vi "HW3_2017_WMA.vi"() -> ()   [LabVIEW 2018]
uses:
  <vilib>/sound2/lvsound2.llb/Sound Output Task ID.ctl
panel:
  in  "shut up":bool
  out "Boolean 3":bool
  out "Boolean 2":bool
  out "Cluster 2":T1
  out "Cluster 3":T1
  out "Cluster 4":T1
  out "Cluster 5":T1
  out "Cluster 6":T1
  out "Cluster 7":T1
  in  "START/STOP/CLEAR":bool
  in  "min":dbl
  in  "hour":dbl
  in  "OK Button":bool
  out "Boolean":bool
  in  "SET ALARM":bool
  out "ALARMING TIME":string
  out "DATE":string
  in  "reinstate":bool
  in  "sec":dbl
  in  "min":dbl
  in  "hour":dbl
  in  "reset":bool
  out "sec":dbl(knob) scale=0.0..60.0
  out "min":dbl(knob) scale=0.0..60.0
  out "hour":dbl(knob) scale=0.0..12.0
  in  "stop":bool
  in  "OK Button 3":bool
  in  "Path 2":path
  out "new picture":picture
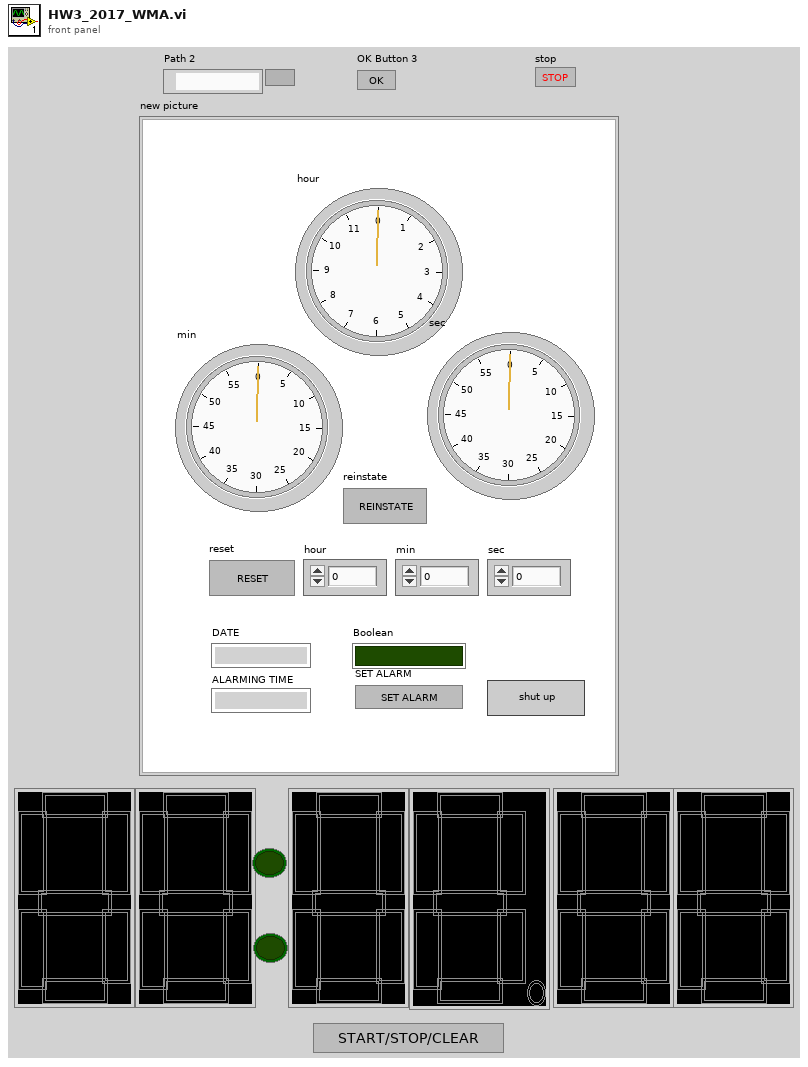
[diagram p1: front panel]
types:
  T1 = cluster{"0":bool, "1":bool, "2":bool, "3":bool, " 4":bool, "5":bool, "6":bool, "p":bool}
  T2 = cluster{"0":bool, "1":bool, "2":bool, "3":bool, " 4":bool, "5":bool, "6":bool, "p":bool}[]
  T3 = typedef "LVDateTimeRec.ctl" = cluster{"fractional second":dbl, "second":i32, "minute":i32, "hour":i32, "day of month":i32, "month":i32, "year":i32, "day of week":i32, "day of year":i32, "DST":i32}
  T4 = typedef "Sound Output Task ID.ctl" = u32
  T5 = typedef "imagedata.ctl" = cluster{"image type":i32, "image depth":i32, "image":u8[], "mask":u8[], "colors":u32[], "Rectangle":cluster{"left":i16, "top":i16, "right":i16, "bottom":i16}}
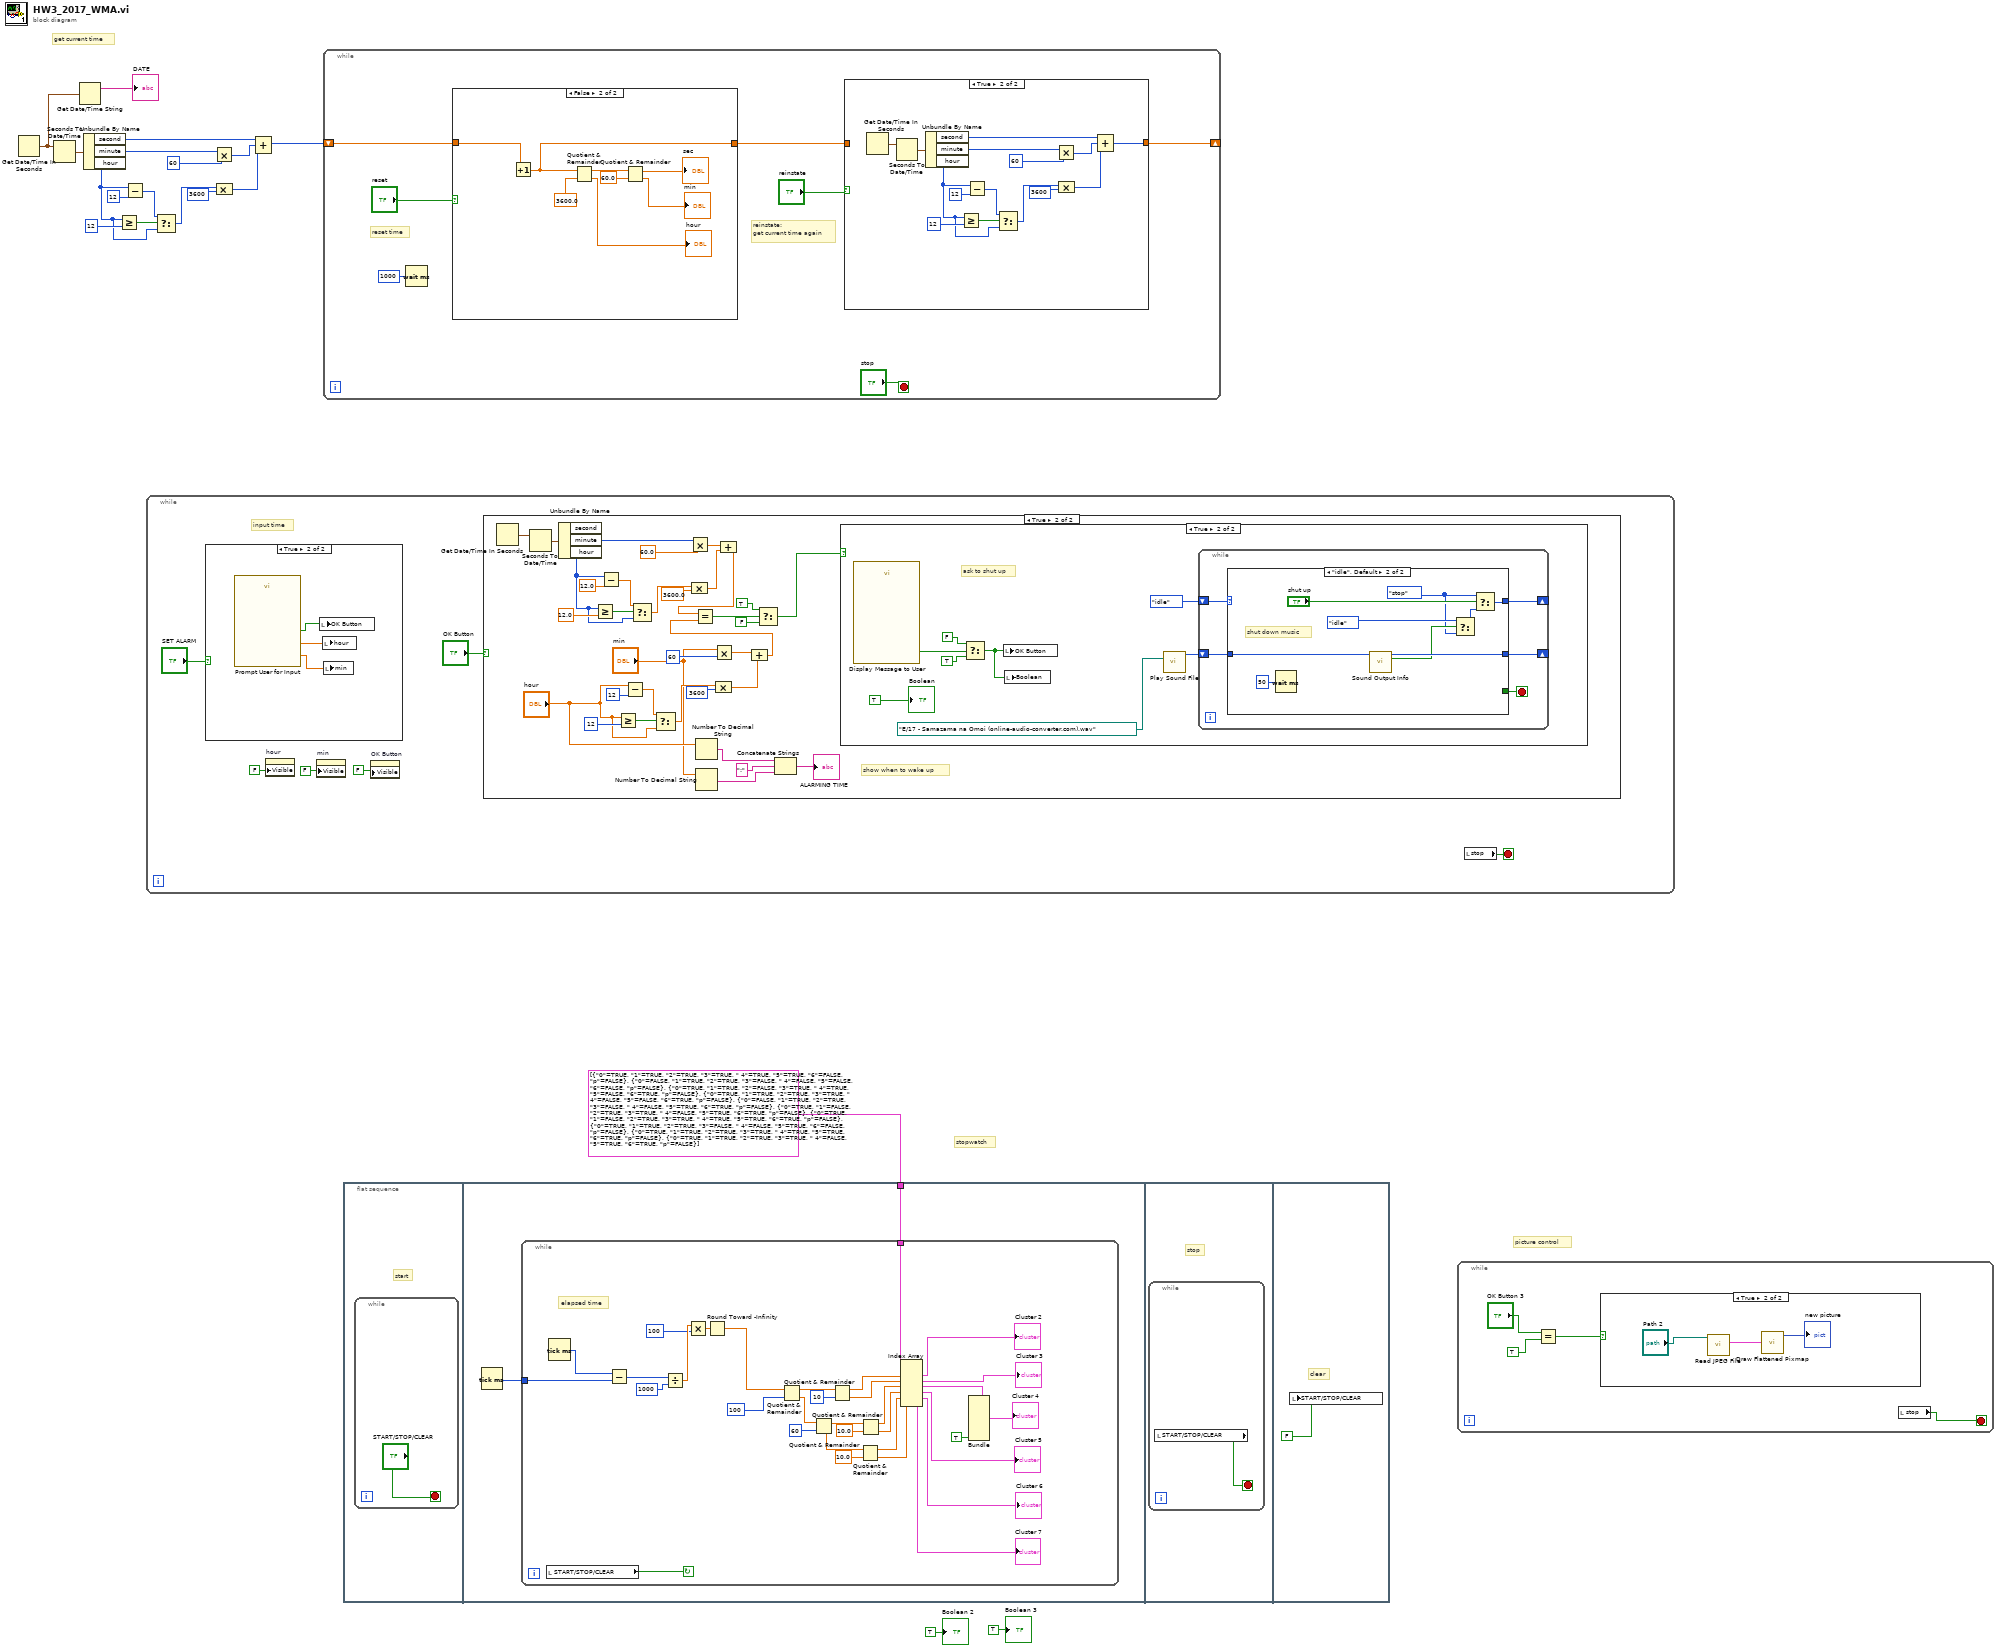
[diagram p0: block diagram]
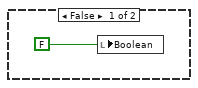
[diagram p4: hidden frame]
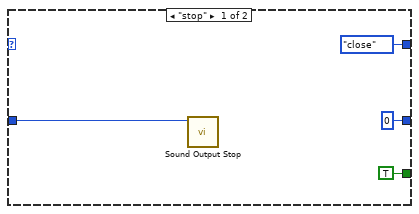
[diagram p5: hidden frame]
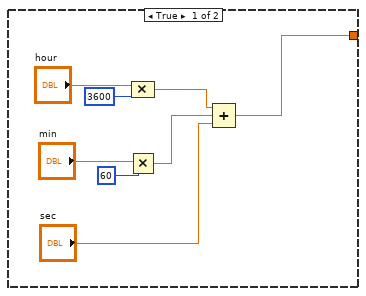
[diagram p8: hidden frame]
diagram:
  # "get current time"
  # "stopwatch"
  # "picture control"
  n1 = Get Date/Time In Seconds() -> (seconds since 1Jan1904=w8:timestamp)
  n2 = Seconds To Date/Time(time stamp (now)=w8) -> (date time rec=w17:T3)  [unwired: 1 in]
  n3 = Get Date/Time String(seconds (now)=w8) -> (date string=→"DATE":string)  [unwired: 2 in, 1 out]
  n4 = Unbundle By Name(w17) -> ("second"=w15:i32, "minute"=w16:i32, "hour"=w10:i32)
  n5 = Greater Or Equal?(x=w10, y=12) -> (x >= y?=w13:bool)
  n6 = Subtract(x=w10, y=12) -> (x-y=w11:i32)
  n7 = while {
    stop <- w21 stop-if-true
    # "input time"
    n8 = case shown="True" "SET ALARM" {
      frame False {
      }
      frame True {
        n9 = call "Prompt User for Input"() -> ("Minute"=w89:dbl, "Hour"=w88:dbl, "OK"=w87:bool)  [unwired: 16 in, 1 out]
        n10 = local write "OK Button"(w87) -> ()
        n11 = local write "hour"(w88) -> ()
        n12 = local write "min"(w89) -> ()
      }
    }
    n13 = property on="hour" class="DigNum (strict)"("Visible"=FALSE) -> ()  [unwired: 2 in, 2 out]
    n14 = property on="min" class="DigNum (strict)"("Visible"=FALSE) -> ()  [unwired: 2 in, 2 out]
    n15 = property on="OK Button" class="Bool (strict)"("Visible"=FALSE) -> ()  [unwired: 2 in, 2 out]
    n16 = case shown="True" "OK Button" {
      frame False {
      }
      frame True {
        # "show when to wake up"
        n17 = Get Date/Time In Seconds() -> (seconds since 1Jan1904=w29:timestamp)
        n18 = Seconds To Date/Time(time stamp (now)=w29) -> (date time rec=w32:T3)  [unwired: 1 in]
        n19 = Unbundle By Name(w32) -> ("minute"=w33:i32, "hour"=w27:i32)  [unwired: 1 out]
        n20 = Greater Or Equal?(x=w27, y=12.0) -> (x >= y?=w35:bool)
        n21 = Subtract(x=w27, y=12.0) -> (x-y=w37:dbl)
        n22 = Greater Or Equal?(x="hour", y=12) -> (x >= y?=w54:bool)
        n23 = Subtract(x="hour", y=12) -> (x-y=w52:dbl)
        n24 = Select(t=w37, s=w35, f=w27) -> (s? t:f=w38:dbl)
        n25 = Select(t=w52, s=w54, f="hour") -> (s? t:f=w51:dbl)
        n26 = Multiply(x=w33, y=60.0) -> (x*y=w39:dbl)
        n27 = Compound Arithmetic op=MULTIPLY(w38, 3600.0) -> (w40:dbl)
        n28 = Number To Decimal String(number="hour") -> (decimal integer string=w46:string)  [unwired: 1 in]
        n29 = Number To Decimal String(number="min") -> (decimal integer string=w44:string)  [unwired: 1 in]
        n30 = Multiply(x="min", y=60) -> (x*y=w57:dbl)
        n31 = Compound Arithmetic op=MULTIPLY(w51, 3600) -> (w56:dbl)
        n32 = Compound Arithmetic op=ADD(w39, w40) -> (w28:dbl)
        n33 = Compound Arithmetic op=ADD(w57, w56) -> (w50:dbl)
        n34 = Equal?(x=w28, y=w50) -> (x = y?=w49:bool)
        n35 = Select(t=TRUE, s=w49, f=FALSE) -> (s? t:f=w26:bool)
        n36 = Concatenate Strings(w46, ":", w44) -> (→"ALARMING TIME":string)
        n37 = case shown="True" w26 {
          frame False {
            n38 = local write "Boolean"(FALSE ("Boolean")) -> ()
          }
          frame True {
            # "ask to shut up"
            n39 = call "Display Message to User"() -> ("OK"=w66:bool)  [unwired: 10 in, 1 out]
            n40 = Select(t=FALSE ("Boolean"), s=w66, f=TRUE) -> (s? t:f=w64:bool)
            n41 = local write "OK Button"(w64) -> ()
            n42 = local write "Boolean"(w64) -> ()
            n43 = call <vilib>:"Play Sound File.vi"("path"=path "E:/17 - Samazama na Omoi (online-audio-converter.com).wav" ("Path")) -> ("task ID"=w62:T4)  [unwired: 9 in, 1 out]
            n44 = while {
              shift-right: [w69] -> _
              shift-left: enum16{"start", "stop", "close", "idle"}."idle" -> [w73]
              shift-right: [w71] -> _
              shift-left: w62 -> [w70]
              stop <- w72 stop-if-true
              n45 = case shown="\"idle\", Default" w73 {
                tunnel: [TRUE _] -> w72
                tunnel: [T4 0 ("task ID") w84] -> w71
                tunnel: w70 -> [w77 w85]
                tunnel: [enum16{"start", "stop", "close", "idle"}."close" w79] -> w69
                frame "stop" {
                  n46 = call <vilib>:"Sound Output Stop.vi"("task ID"=w77) -> ()  [unwired: 9 in, 2 out]
                }
                frame "idle", Default {
                  w78 = enum16{"start", "stop", "close", "idle"}."stop"
                  # "shut down music"
                  n47 = Wait (ms)(milliseconds to wait=u32 50) -> ()  [unwired: 1 out]
                  n48 = call <vilib>:"Sound Output Info.vi"("task ID"=w85) -> ("is playing?"=w83:bool, "task ID out"=w84:T4)  [unwired: 7 in, 2 out]
                  n49 = Select(t=enum16{"start", "stop", "close", "idle"}."idle", s=w83, f=w78) -> (s? t:f=w81:enum16{"start", "stop", "close", "idle"})
                  n50 = Select(t=w78, s="shut up", f=w81) -> (s? t:f=w79:enum16{"start", "stop", "close", "idle"})
                }
              }
            }
            "Boolean" <- TRUE ("Boolean")
          }
        }
      }
    }
    n51 = local read "stop"() -> (w21:bool)
  }
  n52 = Select(t=w11, s=w13, f=w10) -> (s? t:f=w9:i32)
  n53 = Multiply(x=w16, y=60) -> (x*y=w5:i32)
  n54 = Compound Arithmetic op=MULTIPLY(w9, 3600) -> (w4:i32)
  n55 = Compound Arithmetic op=ADD(w15, w5, w4) -> (w7:i32)
  n56 = while {
    shift-right: [w91] -> _
    shift-left: w7 -> [w95]
    stop <- "stop" stop-if-true
    # "reinstate:\nget current time again"
    # "reset time"
    n57 = Wait (ms)(milliseconds to wait=u32 1000) -> ()  [unwired: 1 out]
    n58 = case shown="False" "reset" {
      tunnel: w95 -> [_ w128]
      tunnel: [w113 w121] -> w92
      frame True {
        n59 = Multiply(x="min", y=60) -> (x*y=w115:dbl)
        n60 = Compound Arithmetic op=MULTIPLY("hour", 3600) -> (w116:dbl)
        n61 = Compound Arithmetic op=ADD(w116, w115, "sec") -> (w113:dbl)
      }
      frame False {
        n62 = Increment(x=w128) -> (x+1=w121:dbl)
        n63 = Quotient & Remainder(x=w121, y=3600.0) -> (x-y*floor(x/y)=w126:dbl, floor(x/y)=→"hour":dbl)
        n64 = Quotient & Remainder(x=w126, y=60.0) -> (x-y*floor(x/y)=→"sec":dbl, floor(x/y)=→"min":dbl)
      }
    }
    n65 = case shown="True" "reinstate" {
      tunnel: w92 -> [w97 _]
      tunnel: [w97 w98] -> w91
      frame False {
      }
      frame True {
        n66 = Get Date/Time In Seconds() -> (seconds since 1Jan1904=w109:timestamp)
        n67 = Seconds To Date/Time(time stamp (now)=w109) -> (date time rec=w108:T3)  [unwired: 1 in]
        n68 = Unbundle By Name(w108) -> ("second"=w105:i32, "minute"=w107:i32, "hour"=w100:i32)
        n69 = Greater Or Equal?(x=w100, y=12) -> (x >= y?=w103:bool)
        n70 = Subtract(x=w100, y=12) -> (x-y=w101:i32)
        n71 = Select(t=w101, s=w103, f=w100) -> (s? t:f=w99:i32)
        n72 = Multiply(x=w107, y=60) -> (x*y=w110:i32)
        n73 = Compound Arithmetic op=MULTIPLY(w99, 3600) -> (w106:i32)
        n74 = Compound Arithmetic op=ADD(w105, w110, w106) -> (w98:i32)
      }
    }
  }
  n75 = flat-sequence {
    tunnel: T2 [{"0"=TRUE, "1"=TRUE, "2"=TRUE, "3"=TRUE, " 4"=TRUE, "5"=TRUE, "6"=FALSE, "p"=FALSE}, {"0"=FALSE, "1"=TRUE, "2"=TRUE, "3"=FALSE, " 4"=FALSE, "5"=FALSE, "6"=FALSE, "p"=FALSE}, {"0"=TRUE, "1"=TRUE, "2"=FALSE, "3"=TRUE, " 4"=TRUE, "5"=FALSE, "6"=TRUE, "p"=FALSE}, {"0"=TRUE, "1"=TRUE, "2"=TRUE, "3"=TRUE, " 4"=FALSE, "5"=FALSE, "6"=TRUE, "p"=FALSE}, {"0"=FALSE, "1"=TRUE, "2"=TRUE, "3"=FALSE, " 4"=FALSE, "5"=TRUE, "6"=TRUE, "p"=FALSE}, {"0"=TRUE, "1"=FALSE, "2"=TRUE, "3"=TRUE, " 4"=FALSE, "5"=TRUE, "6"=TRUE, "p"=FALSE}, {"0"=TRUE, "1"=FALSE, "2"=TRUE, "3"=TRUE, " 4"=TRUE, "5"=TRUE, "6"=TRUE, "p"=FALSE}, {"0"=TRUE, "1"=TRUE, "2"=TRUE, "3"=FALSE, " 4"=FALSE, "5"=TRUE, "6"=FALSE, "p"=FALSE}, {"0"=TRUE, "1"=TRUE, "2"=TRUE, "3"=TRUE, " 4"=TRUE, "5"=TRUE, "6"=TRUE, "p"=FALSE}, {"0"=TRUE, "1"=TRUE, "2"=TRUE, "3"=TRUE, " 4"=FALSE, "5"=TRUE, "6"=TRUE, "p"=FALSE}] -> [w130]
    frame #0 {
      # "start"
      n76 = while {
        stop <- "START/STOP/CLEAR" stop-if-true
      }
    }
    frame #1 {
      n77 = Tick Count (ms)() -> (millisecond timer value=w131:u32)
      n78 = while {
        tunnel: w131 -> [w163]
        tunnel: w130 -> [w145]
        stop <- w160 continue-if-true
        # "elapsed time"
        n79 = local read "START/STOP/CLEAR"() -> (w160:bool)
        n80 = Tick Count (ms)() -> (millisecond timer value=w164:u32)
        n81 = Subtract(x=w164, y=w163) -> (x-y=w162:u32)
        n82 = Divide(x=w162, y=1000) -> (x/y=w159:dbl)
        n83 = Multiply(x=w159, y=100) -> (x*y=w157:dbl)
        n84 = Round Toward -Infinity(1:w157) -> (0:w144:dbl)
        n85 = Quotient & Remainder(x=w144, y=100) -> (x-y*floor(x/y)=w151:dbl, floor(x/y)=w141:dbl)
        n86 = Quotient & Remainder(x=w141, y=60) -> (x-y*floor(x/y)=w138:dbl, floor(x/y)=w134:dbl)
        n87 = Quotient & Remainder(x=w151, y=10) -> (x-y*floor(x/y)=w152:dbl, floor(x/y)=w153:dbl)
        n88 = Quotient & Remainder(x=w134, y=10.0) -> (x-y*floor(x/y)=w133:dbl, floor(x/y)=w132:dbl)
        n89 = Quotient & Remainder(x=w138, y=10.0) -> (x-y*floor(x/y)=w137:dbl, floor(x/y)=w136:dbl)
        n90 = Index Array(array=w145, index #1=w152, index #2=w153, index #3=w137, index #4=w136, index #5=w133, index #6=w132) -> (element #1=→"Cluster 2":T1, element #2=→"Cluster 3":T1, element #3=w154:T1, element #4=→"Cluster 5":T1, element #5=→"Cluster 6":T1, element #6=→"Cluster 7":T1)
        n91 = Bundle(cluster=w154, "p"=TRUE) -> (→"Cluster 4":T1)  [unwired: 7 in]
      }
    }
    frame #2 {
      # "stop"
      n92 = while {
        stop <- w165 stop-if-true
        n93 = local read "START/STOP/CLEAR"() -> (w165:bool)
      }
    }
    frame #3 {
      # "clear"
      n94 = local write "START/STOP/CLEAR"(FALSE ("OK Button")) -> ()
    }
  }
  n95 = while {
    stop <- w167 stop-if-true
    n96 = Equal?(x="OK Button 3", y=TRUE) -> (x = y?=w168:bool)
    n97 = case shown="True" w168 {
      frame False {
      }
      frame True {
        n98 = call <vilib>:"Read JPEG File.vi"("path to JPEG file"="Path 2") -> ("image data"=w172:T5)  [unwired: 8 in, 2 out]
        n99 = call <vilib>:"Draw Flattened Pixmap.vi"("image data"=w172) -> ("new picture"=→"new picture":picture)  [unwired: 8 in]
      }
    }
    n100 = local read "stop"() -> (w167:bool)
  }
  "Boolean 2" <- TRUE ("Boolean")
  "Boolean 3" <- TRUE ("Boolean 2")
